vi "Edwards PV convert.vi"(11 "error in":errorcluster) -> (0 "error out":errorcluster, 2 "Output Variable 2":dbl format="%#_3e", 3 "Output Variable 1":dbl format="%#_3e")   [LabVIEW 2023]
uses:
  <vilib>/Analysis/baseanly.llb/Mean (DBL).vi
  <vilib>/Analysis/NI_AALBase.lvlib
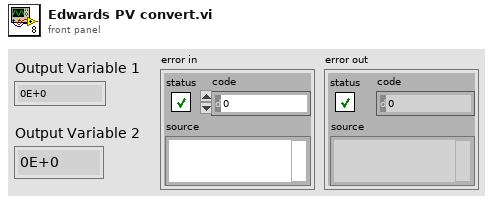
[diagram p1: front panel]
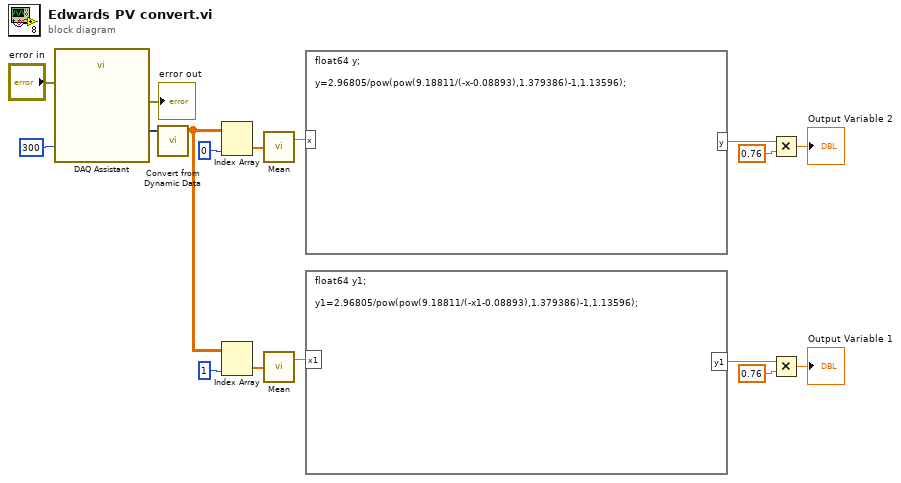
[diagram p0: block diagram]
diagram:
  n1 = call "DAQ Assistant"("number of samples"=300, "error in"="error in") -> ("data"=w10:dynamicdata, "error out"=→"error out":errorcluster)  [unwired: 15 in, 1 out]
  n2 = call "Convert from Dynamic Data"("Dynamic Data Type"=w10) -> ("Array"=w14:dbl[][])  [unwired: 3 in]
  n3 = Index Array(array=w14, index (col)=0 ("disabled index (col)")) -> (element=w12:dbl[])  [unwired: 1 in]
  n4 = Index Array(array=w14, index (col)=1 ("disabled index (col)")) -> (element=w15:dbl[])  [unwired: 1 in]
  n5 = call-poly <vilib>:"Mean.vi"("X"=w12) -> ("mean"=w16:dbl)  [unwired: 1 out]
  n6 = call-poly <vilib>:"Mean.vi"("X"=w15) -> ("mean"=w17:dbl)  [unwired: 1 out]
  n7 = formula code="float64 y;\n\ny=2.96805/pow(pow(9.18811/(-x-0.08893),1.379386)-1,1.13596);"("x"=w16) -> ("y"=w3:dbl)
  n8 = formula code="float64 y1;\n\ny1=2.96805/pow(pow(9.18811/(-x1-0.08893),1.379386)-1,1.13596);"("x1"=w17) -> ("y1"=w8:dbl)
  n9 = Multiply(x=w3, y=0.76) -> (x*y=→"Output Variable 2":dbl)
  n10 = Multiply(x=w8, y=0.76) -> (x*y=→"Output Variable 1":dbl)
